vi "IVCharacterization.vi"() -> ()   [LabVIEW 2020]
panel:
  in  "循环":bool
  in  "参数值":dbl[](array[numeric])
  in  "负向扫描":bool
  in  "正向扫描":bool
  out "参数":string[](array[string])
  in  "Y轴":u16(ring)=2 items=["Time", "Voltage", "Current", "Real V"]
  in  "X轴":u16(ring)=1 items=["Time", "Voltage", "Current", "Real V"]
  out "XY图":picture
  in  "log":bool
  in  "缓冲区数据内容":u16(ring) items=["SET", "RESET", "TIME", "PSET", "PRESET"]
  out "缓存数据":bool
  in  "清除缓存数据":bool
  in  "功能选择":u16(ring)=1 items=["I-V扫描", "脉冲测试", "维持时间"]
  in  "4-wire":bool
  in  "自行输入nplc":bool
  in  "时序优先":bool
  in  "测试人员":string
  in  "衬底":string(combo)
  in  "阻变物质":string(combo)
  in  "保存数据":bool
  in  "停止":bool
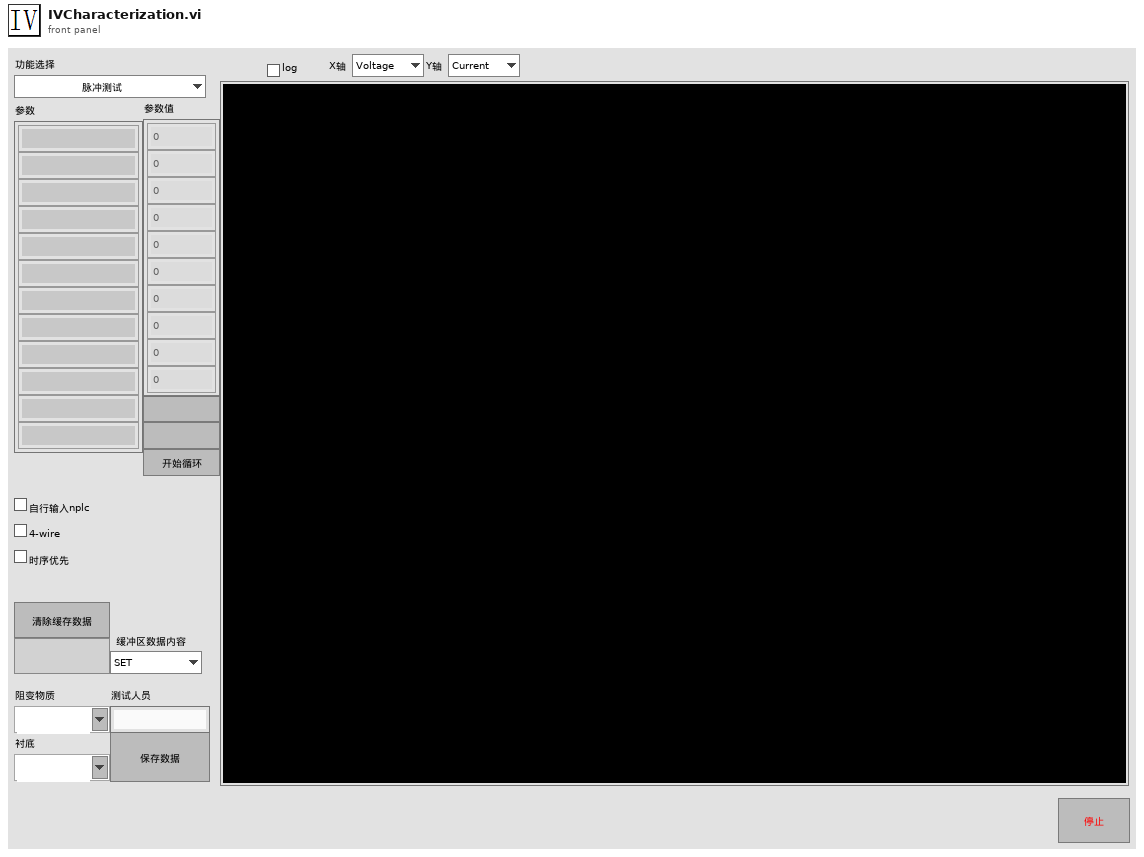
[diagram p1: front panel]
types:
  T1 = cluster{"nplc":dbl, "时序优先":bool, "时间点(ms)":dbl, "电压改变量":dbl, "极限电流(mA)":dbl, "扫描电压(V)":dbl, "4-wire ":bool}
  T2 = cluster{"nplc":dbl, "脉冲宽度(ms)":dbl, "读取电压":dbl, "极限电流(mA)":dbl, "脉冲电压(V)":dbl, "4-wire":bool, "读取次数":dbl}
  T3 = cluster{"nplc":dbl, "4-wire":bool, "读取间隔(ms)":dbl, "读取数量":dbl, "极限电流(mA)":dbl, "读取电压(V)":dbl}
  T4 = cluster{"测试人员":string, "阻变物质":string, "衬底":string}
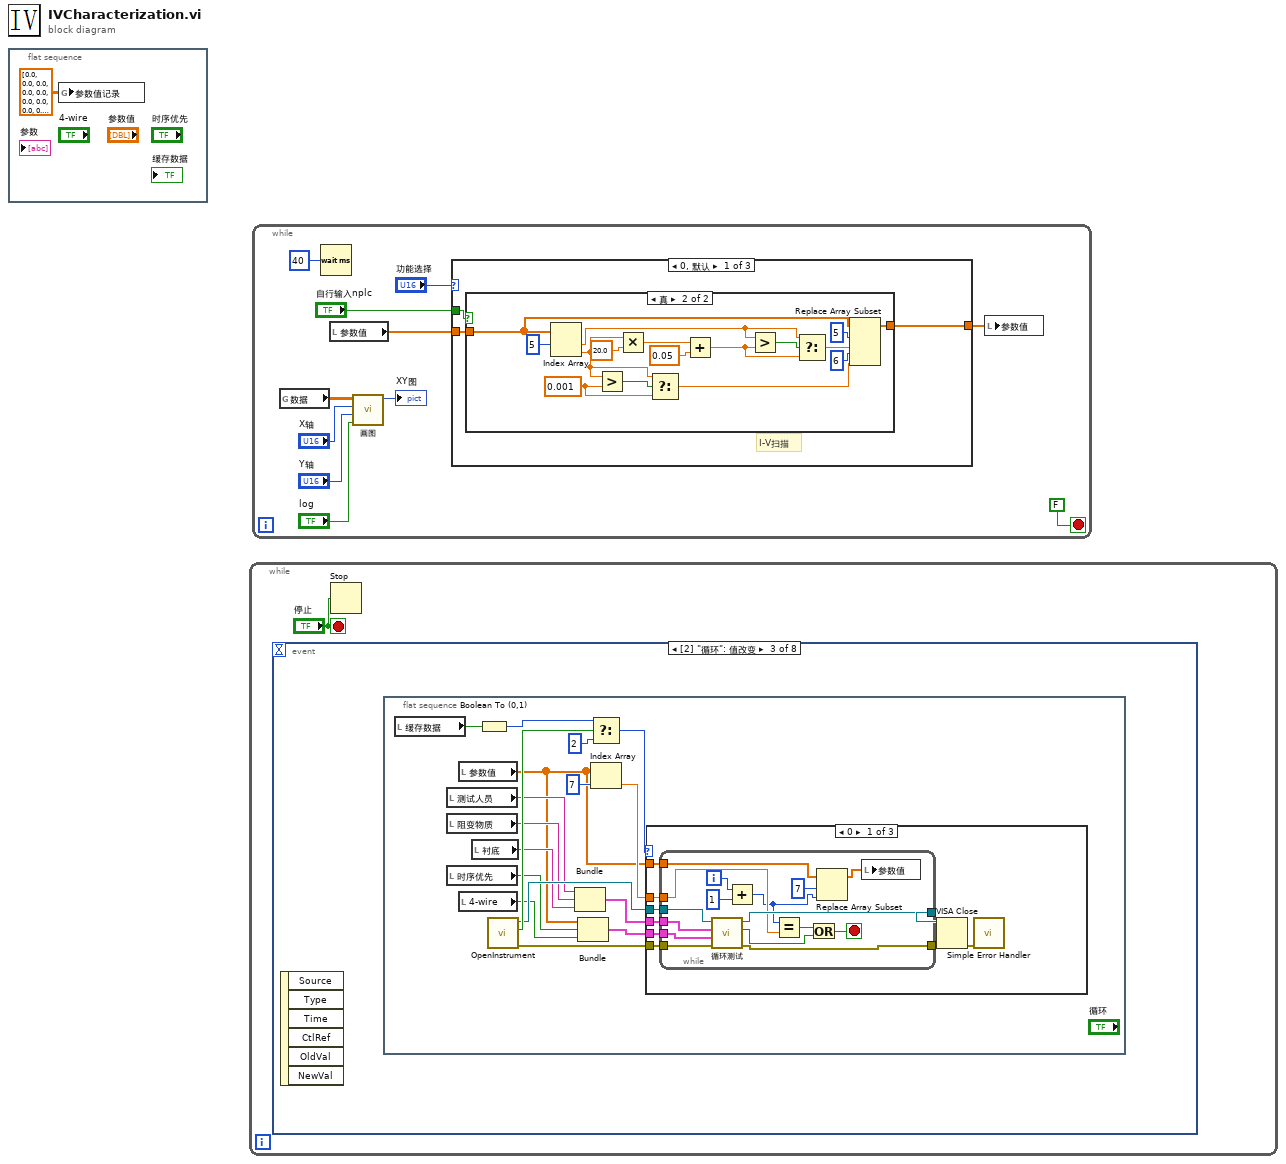
[diagram p0: block diagram]
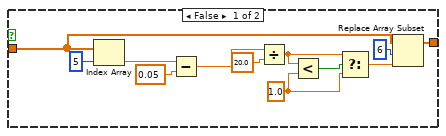
[diagram p2: hidden frame]
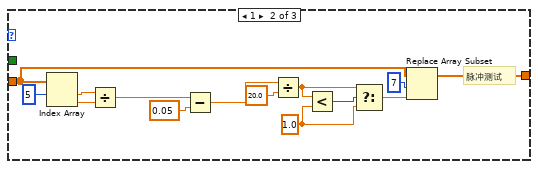
[diagram p3: hidden frame]
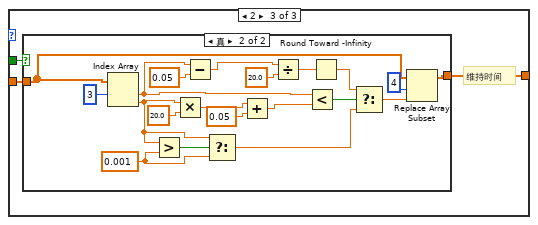
[diagram p4: hidden frame]
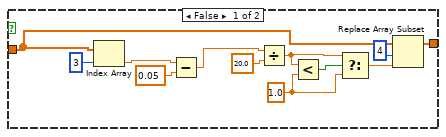
[diagram p5: hidden frame]
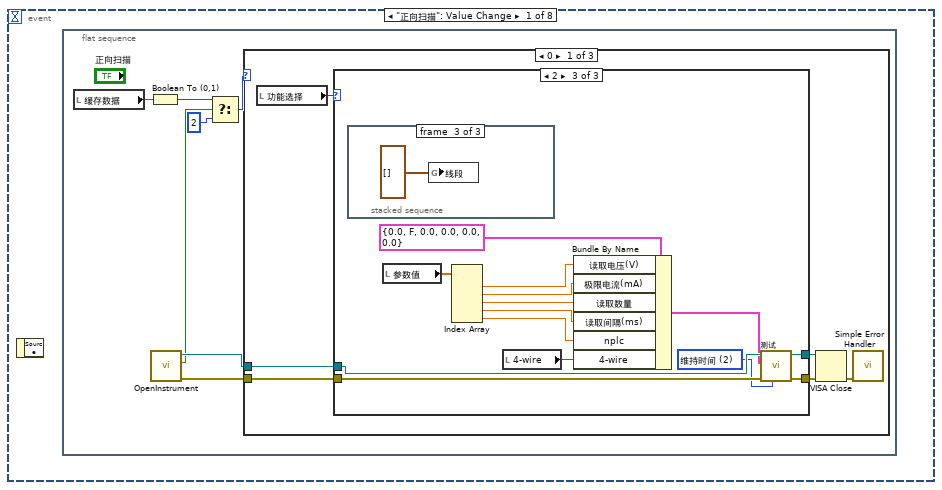
[diagram p6: hidden frame]
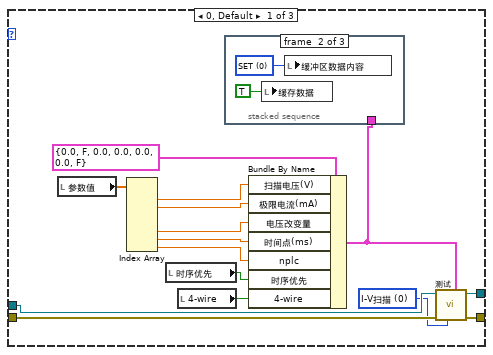
[diagram p7: hidden frame]
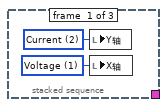
[diagram p8: hidden frame]
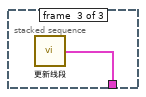
[diagram p9: hidden frame]
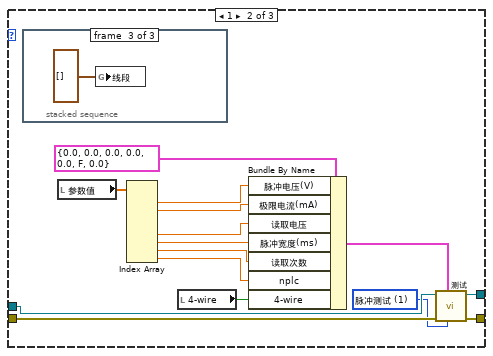
[diagram p10: hidden frame]
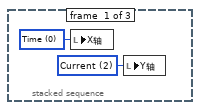
[diagram p11: hidden frame]
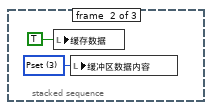
[diagram p12: hidden frame]
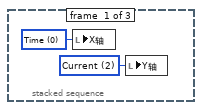
[diagram p13: hidden frame]
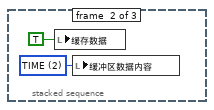
[diagram p14: hidden frame]
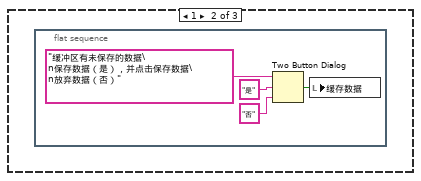
[diagram p15: hidden frame]
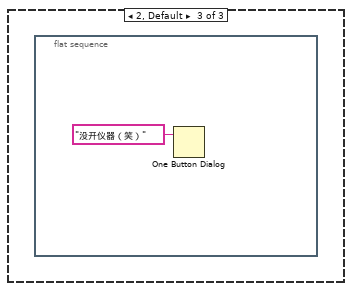
[diagram p16: hidden frame]
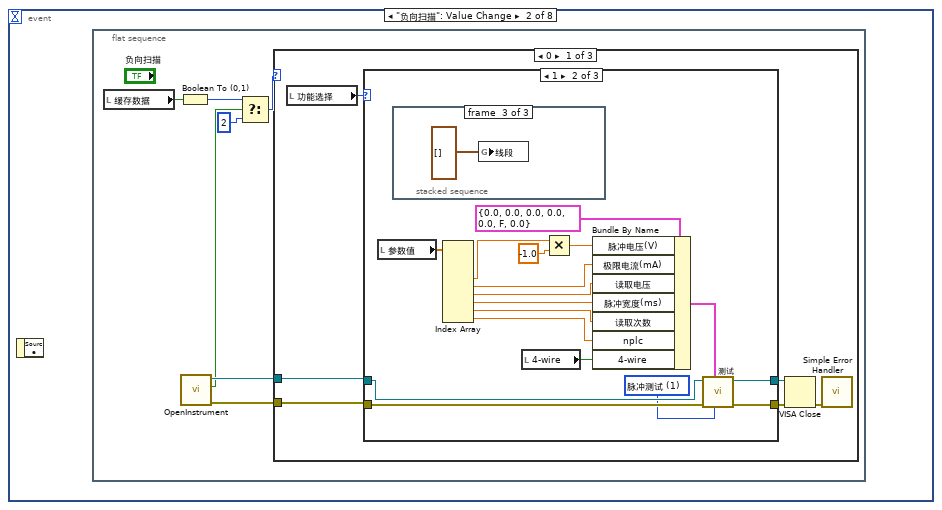
[diagram p17: hidden frame]
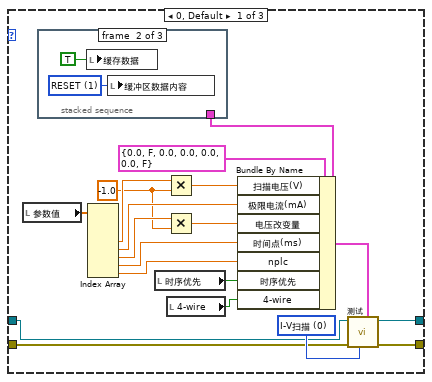
[diagram p18: hidden frame]
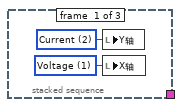
[diagram p19: hidden frame]
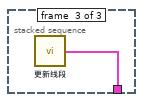
[diagram p20: hidden frame]
diagram:
  n1 = flat-sequence {
    frame #0 {
      n2 = global write "Global variable.vi" "参数值记录"(dbl[][] [[0.0, 0.0, 0.0, 0.0, 0.0, 0.0, 0.0, 0.0, 0.0, 0.0, 0.0, 0.0, 0.0, 0.0, 0.0, 0.0, 0.0, 0.0], [0.0, 0.0, 0.0, 0.0, 0.0, 0.0, 0.0, 0.0, 0.0, 0.0, 0.0, 0.0, 0.0, 0.0, 0.0, 0.0, 0.0, 0.0], [0.0, 0.0, 0.0, 0.0, 0.0, 0.0, 0.0, 0.0, 0.0, 0.0, 0.0, 0.0, 0.0, 0.0, 0.0, 0.0, 0.0, 0.0], [0.0, 0.0, 0.0, 0.0, 0.0, 0.0, 0.0, 0.0, 0.0, 0.0, 0.0, 0.0, 0.0, 0.0, 0.0, 0.0, 0.0, 0.0], [0.0, 0.0, 0.0, 0.0, 0.0, 0.0, 0.0, 0.0, 0.0, 0.0, 0.0, 0.0, 0.0, 0.0, 0.0, 0.0, 0.0, 0.0], [0.0, 0.0, 0.0, 0.0, 0.0, 0.0, 0.0, 0.0, 0.0, 0.0, 0.0, 0.0, 0.0, 0.0, 0.0, 0.0, 0.0, 0.0], [0.0, 0.0, 0.0, 0.0, 0.0, 0.0, 0.0, 0.0, 0.0, 0.0, 0.0, 0.0, 0.0, 0.0, 0.0, 0.0, 0.0, 0.0], [0.0, 0.0, 0.0, 0.0, 0.0, 0.0, 0.0, 0.0, 0.0, 0.0, 0.0, 0.0, 0.0, 0.0, 0.0, 0.0, 0.0, 0.0], [0.0, 0.0, 0.0, 0.0, 0.0, 0.0, 0.0, 0.0, 0.0, 0.0, 0.0, 0.0, 0.0, 0.0, 0.0, 0.0, 0.0, 0.0], [0.0, 0.0, 0.0, 0.0, 0.0, 0.0, 0.0, 0.0, 0.0, 0.0, 0.0, 0.0, 0.0, 0.0, 0.0, 0.0, 0.0, 0.0], [0.0, 0.0, 0.0, 0.0, 0.0, 0.0, 0.0, 0.0, 0.0, 0.0, 0.0, 0.0, 0.0, 0.0, 0.0, 0.0, 0.0, 0.0], [0.0, 0.0, 0.0, 0.0, 0.0, 0.0, 0.0, 0.0, 0.0, 0.0, 0.0, 0.0, 0.0, 0.0, 0.0, 0.0, 0.0, 0.0], [0.0, 0.0, 0.0, 0.0, 0.0, 0.0, 0.0, 0.0, 0.0, 0.0, 0.0, 0.0, 0.0, 0.0, 0.0, 0.0, 0.0, 0.0], [0.0, 0.0, 0.0, 0.0, 0.0, 0.0, 0.0, 0.0, 0.0, 0.0, 0.0, 0.0, 0.0, 0.0, 0.0, 0.0, 0.0, 0.0], [0.0, 0.0, 0.0, 0.0, 0.0, 0.0, 0.0, 0.0, 0.0, 0.0, 0.0, 0.0, 0.0, 0.0, 0.0, 0.0, 0.0, 0.0], [0.0, 0.0, 0.0, 0.0, 0.0, 0.0, 0.0, 0.0, 0.0, 0.0, 0.0, 0.0, 0.0, 0.0, 0.0, 0.0, 0.0, 0.0], [0.0, 0.0, 0.0, 0.0, 0.0, 0.0, 0.0, 0.0, 0.0, 0.0, 0.0, 0.0, 0.0, 0.0, 0.0, 0.0, 0.0, 0.0]]) -> ()
    }
  }
  n3 = while {
    stop <- "停止" stop-if-true
    n4 = event "事件结构" shown="[2] \"循环\": 值改变" {
      selector: _ -> [_ _ _ _ _ _ _ _]
      dyn-events: _ -> [_ _ _ _ _ _ _ _]
      timeout: _ -> [_ _ _ _ _ _ _ _]
      event "正向扫描": Value Change {
        n5 = event-data() -> ()  [unwired: 1 in, 1 out]
        n6 = flat-sequence {
          frame #0 {
            n7 = local read "缓存数据"() -> (w7:bool)
            n8 = Boolean To (0,1)(Boolean=w7) -> (0, 1=w5:i16)
            n9 = call "OpenInstrument.vi"() -> ("错误输出"=w9:errorcluster, "仪器存在"=w6:bool, "VISA资源名称输出"=w8:refnum<visa-resource-name>)  [unwired: 9 in]
            n10 = Select(t=w5, s=w6, f=i16 2) -> (s? t:f=w4:i16)
            n11 = case shown="0" w4 {
              tunnel: w9 -> [w11 _ _]
              tunnel: w8 -> [w10 _ _]
              frame 0 {
                n12 = local read "功能选择"() -> (w15:u16)
                n13 = case shown="2" w15 {
                  tunnel: w10 -> [w30 w50 w66]
                  tunnel: [w29 w48 w67] -> w12
                  tunnel: [w28 w47 w68] -> w13
                  tunnel: w11 -> [w27 w49 w69]
                  frame 0, Default {
                    w17 = u16 0 items=["I-V扫描", "脉冲测试", "维持时间"] ("功能选择")
                    n14 = local read "参数值"() -> (w23:dbl[])
                    n15 = Index Array(array=w23) -> (element #1=w22:dbl, element #2=w21:dbl, element #5=w20:dbl, element #6=w19:dbl, element #7=w18:dbl)  [unwired: 7 in, 2 out]
                    n16 = local read "时序优先"() -> (w25:bool)
                    n17 = local read "4-wire"() -> (w24:bool)
                    n18 = Bundle By Name(cluster=T1 {"nplc"=0.0, "时序优先"=FALSE, "时间点(ms)"=0.0, "电压改变量"=0.0, "极限电流(mA)"=0.0, "扫描电压(V)"=0.0, "4-wire "=FALSE} ("参数"), "扫描电压(V)"=w22, "极限电流(mA)"=w21, "电压改变量"=w20, "时间点(ms)"=w19, "nplc"=w18, "时序优先"=w25, "4-wire"=w24) -> (w16:T1)
                    n19 = stacked-sequence {
                      tunnel: w16 -> [_ _ w35]
                      frame #0 {
                        w31 = u16 2 items=["Time", "Voltage", "Current"] ("X轴")
                        w32 = u16 1 items=["Time", "Voltage", "Current"] ("X轴")
                        n20 = local write "Y轴"(w31) -> ()
                        n21 = local write "X轴"(w32) -> ()
                      }
                      frame #1 {
                        w34 = u16 0 items=["SET", "RESET", "TIME"] ("缓冲区数据内容")
                        n22 = local write "缓存数据"(TRUE) -> ()
                        n23 = local write "缓冲区数据内容"(w34) -> ()
                      }
                      frame #2 {
                        n24 = call "更新线段.vi"("参数"=w35) -> ()
                      }
                    }
                    n25 = call "测试.vi"("I-V扫描"=w16, "功能选择"=w17, "错误输入"=w27, "VISA资源名称"=w30) -> ("错误输出"=w28:errorcluster, "VISA资源名称输出"=w29:refnum<visa-resource-name>)  [unwired: 6 in]
                  }
                  frame 1 {
                    w37 = u16 1 items=["I-V扫描", "脉冲测试", "维持时间"] ("功能选择")
                    n26 = stacked-sequence {
                      frame #0 {
                        w51 = u16 2 items=["Time", "Voltage", "Current"] ("X轴")
                        w52 = u16 0 items=["Time", "Voltage", "Current"] ("X轴")
                        n27 = local write "X轴"(w52) -> ()
                        n28 = local write "Y轴"(w51) -> ()
                      }
                      frame #1 {
                        w54 = u16 3 items=["SET", "RESET", "TIME", "Pset", "Preset"] ("缓冲区数据内容")
                        n29 = local write "缓存数据"(TRUE ("缓存数据")) -> ()
                        n30 = local write "缓冲区数据内容"(w54) -> ()
                      }
                      frame #2 {
                        n31 = global write "Global variable.vi" "线段"(cluster{i32, i32}[] [] ("线段")) -> ()
                      }
                    }
                    n32 = local read "参数值"() -> (w44:dbl[])
                    n33 = Index Array(array=w44) -> (element #1=w43:dbl, element #2=w42:dbl, element #5=w41:dbl, element #6=w40:dbl, element #7=w39:dbl, element #8=w38:dbl)  [unwired: 8 in, 2 out]
                    n34 = local read "4-wire"() -> (w45:bool)
                    n35 = Bundle By Name(cluster=T2 {"nplc"=0.0, "脉冲宽度(ms)"=0.0, "读取电压"=0.0, "极限电流(mA)"=0.0, "脉冲电压(V)"=0.0, "4-wire"=FALSE, "读取次数"=0.0} ("脉冲测试"), "脉冲电压(V)"=w43, "极限电流(mA)"=w42, "读取电压"=w41, "脉冲宽度(ms)"=w40, "读取次数"=w39, "nplc"=w38, "4-wire"=w45) -> (w36:T2)
                    n36 = call "测试.vi"("功能选择"=w37, "脉冲测试"=w36, "错误输入"=w49, "VISA资源名称"=w50) -> ("错误输出"=w47:errorcluster, "VISA资源名称输出"=w48:refnum<visa-resource-name>)  [unwired: 6 in]
                  }
                  frame 2 {
                    w56 = u16 2 items=["I-V扫描", "脉冲测试", "维持时间"] ("功能选择")
                    n37 = stacked-sequence {
                      frame #0 {
                        w70 = u16 2 items=["Time", "Voltage", "Current"] ("X轴")
                        w71 = u16 0 items=["Time", "Voltage", "Current"] ("X轴")
                        n38 = local write "X轴"(w71) -> ()
                        n39 = local write "Y轴"(w70) -> ()
                      }
                      frame #1 {
                        w73 = u16 2 items=["SET", "RESET", "TIME"] ("缓冲区数据内容")
                        n40 = local write "缓存数据"(TRUE ("正标记")) -> ()
                        n41 = local write "缓冲区数据内容"(w73) -> ()
                      }
                      frame #2 {
                        n42 = global write "Global variable.vi" "线段"(cluster{i32, i32}[] [] ("线段")) -> ()
                      }
                    }
                    n43 = local read "参数值"() -> (w65:dbl[])
                    n44 = Index Array(array=w65) -> (element #1=w63:dbl, element #2=w62:dbl, element #3=w61:dbl, element #4=w60:dbl, element #5=w59:dbl)  [unwired: 5 in]
                    n45 = local read "4-wire"() -> (w58:bool)
                    n46 = Bundle By Name(cluster=T3 {"nplc"=0.0, "4-wire"=FALSE, "读取间隔(ms)"=0.0, "读取数量"=0.0, "极限电流(mA)"=0.0, "读取电压(V)"=0.0} ("参数"), "读取电压(V)"=w63, "极限电流(mA)"=w62, "读取数量"=w61, "读取间隔(ms)"=w60, "nplc"=w59, "4-wire"=w58) -> (w57:T3)
                    n47 = call "测试.vi"("功能选择"=w56, "错误输入"=w69, "维持时间"=w57, "VISA资源名称"=w66) -> ("错误输出"=w68:errorcluster, "VISA资源名称输出"=w67:refnum<visa-resource-name>)  [unwired: 6 in]
                  }
                }
                n48 = VISA Close(VISA resource name=w12, error in (no error)=w13) -> (error out=w14:errorcluster)
                n49 = call <vilib>:"Simple Error Handler.vi"("error in (no error)"=w14) -> ()  [unwired: 4 in, 5 out]
              }
              frame 1 {
                n50 = flat-sequence {
                  frame #0 {
                    n51 = Two Button Dialog(message="缓冲区有未保存的数据\n保存数据（是），并点击保存数据\n放弃数据（否）" ("消息"), 1:"否" ("F按钮名称（“取消”）"), 2:"是" ("T按钮名称（“确定”）")) -> (T button?=w75:bool)
                    n52 = local write "缓存数据"(w75) -> ()
                  }
                }
              }
              frame 2, Default {
                n53 = flat-sequence {
                  frame #0 {
                    n54 = One Button Dialog(message="没开仪器（笑）" ("消息")) -> ()  [unwired: 1 in, 1 out]
                  }
                }
              }
            }
          }
        }
      }
      event "负向扫描": Value Change {
        n55 = event-data() -> ()  [unwired: 1 in, 1 out]
        n56 = flat-sequence {
          frame #0 {
            n57 = local read "缓存数据"() -> (w81:bool)
            n58 = Boolean To (0,1)(Boolean=w81) -> (0, 1=w84:i16)
            n59 = call "OpenInstrument.vi"() -> ("错误输出"=w86:errorcluster, "仪器存在"=w82:bool, "VISA资源名称输出"=w85:refnum<visa-resource-name>)  [unwired: 9 in]
            n60 = Select(t=w84, s=w82, f=i16 2) -> (s? t:f=w80:i16)
            n61 = case shown="0" w80 {
              tunnel: w86 -> [w88 _ _]
              tunnel: w85 -> [w87 _ _]
              frame 0 {
                n62 = local read "功能选择"() -> (w92:u16)
                n63 = case shown="1" w92 {
                  tunnel: w87 -> [w94 w129 w139]
                  tunnel: [w110 w127 w139] -> w89
                  tunnel: [w109 w126 w138] -> w90
                  tunnel: w88 -> [w95 w128 w138]
                  frame 0, Default {
                    w97 = -1.0 ("y")
                    w96 = u16 0 items=["I-V扫描", "脉冲测试", "维持时间"] ("功能选择")
                    n64 = local read "参数值"() -> (w103:dbl[])
                    n65 = Index Array(array=w103) -> (element #3=w102:dbl, element #4=w101:dbl, element #5=w100:dbl, element #6=w99:dbl, element #7=w98:dbl)  [unwired: 7 in, 2 out]
                    n66 = local read "时序优先"() -> (w107:bool)
                    n67 = Multiply(x=w102, y=w97) -> (x*y=w105:dbl)
                    n68 = Multiply(x=w100, y=w97) -> (x*y=w104:dbl)
                    n69 = local read "4-wire"() -> (w106:bool)
                    n70 = Bundle By Name(cluster=T1 {"nplc"=0.0, "时序优先"=FALSE, "时间点(ms)"=0.0, "电压改变量"=0.0, "极限电流(mA)"=0.0, "扫描电压(V)"=0.0, "4-wire "=FALSE} ("参数"), "扫描电压(V)"=w105, "极限电流(mA)"=w101, "电压改变量"=w104, "时间点(ms)"=w99, "nplc"=w98, "时序优先"=w107, "4-wire"=w106) -> (w93:T1)
                    n71 = stacked-sequence {
                      tunnel: w93 -> [_ _ w115]
                      frame #0 {
                        w111 = u16 2 items=["Time", "Voltage", "Current"] ("X轴")
                        w112 = u16 1 items=["Time", "Voltage", "Current"] ("X轴")
                        n72 = local write "Y轴"(w111) -> ()
                        n73 = local write "X轴"(w112) -> ()
                      }
                      frame #1 {
                        w114 = u16 1 items=["SET", "RESET", "TIME"] ("缓冲区数据内容")
                        n74 = local write "缓存数据"(TRUE) -> ()
                        n75 = local write "缓冲区数据内容"(w114) -> ()
                      }
                      frame #2 {
                        n76 = call "更新线段.vi"("参数"=w115) -> ()
                      }
                    }
                    n77 = call "测试.vi"("I-V扫描"=w93, "功能选择"=w96, "错误输入"=w95, "VISA资源名称"=w94) -> ("错误输出"=w109:errorcluster, "VISA资源名称输出"=w110:refnum<visa-resource-name>)  [unwired: 6 in]
                  }
                  frame 1 {
                    w117 = u16 1 items=["I-V扫描", "脉冲测试", "维持时间"] ("功能选择")
                    n78 = local read "参数值"() -> (w130:dbl[])
                    n79 = stacked-sequence {
                      frame #0 {
                        w133 = u16 2 items=["Time", "Voltage", "Current"] ("X轴")
                        w134 = u16 0 items=["Time", "Voltage", "Current"] ("X轴")
                        n80 = local write "X轴"(w134) -> ()
                        n81 = local write "Y轴"(w133) -> ()
                      }
                      frame #1 {
                        w136 = u16 4 items=["SET", "RESET", "TIME", "Pset", "Preset"] ("缓冲区数据内容")
                        n82 = local write "缓存数据"(TRUE ("缓存数据")) -> ()
                        n83 = local write "缓冲区数据内容"(w136) -> ()
                      }
                      frame #2 {
                        n84 = global write "Global variable.vi" "线段"(cluster{i32, i32}[] [] ("线段")) -> ()
                      }
                    }
                    n85 = Index Array(array=w130) -> (element #3=w123:dbl, element #4=w122:dbl, element #5=w121:dbl, element #6=w120:dbl, element #7=w119:dbl, element #8=w118:dbl)  [unwired: 8 in, 2 out]
                    n86 = local read "4-wire"() -> (w131:bool)
                    n87 = Multiply(x=w123, y=-1.0) -> (x*y=w124:dbl)
                    n88 = Bundle By Name(cluster=T2 {"nplc"=0.0, "脉冲宽度(ms)"=0.0, "读取电压"=0.0, "极限电流(mA)"=0.0, "脉冲电压(V)"=0.0, "4-wire"=FALSE, "读取次数"=0.0} ("脉冲测试"), "脉冲电压(V)"=w124, "极限电流(mA)"=w122, "读取电压"=w121, "脉冲宽度(ms)"=w120, "读取次数"=w119, "nplc"=w118, "4-wire"=w131) -> (w116:T2)
                    n89 = call "测试.vi"("功能选择"=w117, "脉冲测试"=w116, "错误输入"=w128, "VISA资源名称"=w129) -> ("错误输出"=w126:errorcluster, "VISA资源名称输出"=w127:refnum<visa-resource-name>)  [unwired: 6 in]
                  }
                  frame 2 {
                  }
                }
                n90 = VISA Close(VISA resource name=w89, error in (no error)=w90) -> (error out=w91:errorcluster)
                n91 = call <vilib>:"Simple Error Handler.vi"("error in (no error)"=w91) -> ()  [unwired: 4 in, 5 out]
              }
              frame 1 {
                n92 = flat-sequence {
                  frame #0 {
                    n93 = Two Button Dialog(message="缓冲区有未保存的数据\n保存数据（是），并点击保存数据\n放弃数据（否）" ("消息"), 1:"否" ("F按钮名称（“取消”）"), 2:"是" ("T按钮名称（“确定”）")) -> (T button?=w140:bool)
                    n94 = local write "缓存数据"(w140) -> ()
                  }
                }
              }
              frame 2, Default {
                n95 = flat-sequence {
                  frame #0 {
                    n96 = One Button Dialog(message="没开仪器（笑）" ("消息")) -> ()  [unwired: 1 in, 1 out]
                  }
                }
              }
            }
          }
        }
      }
      event "循环": Value Change {
        n97 = event-data() -> ()  [unwired: 1 in, 6 out]
        n98 = flat-sequence {
          frame #0 {
            n99 = local read "缓存数据"() -> (w158:bool)
            n100 = local read "测试人员"() -> (w154:string)
            n101 = local read "阻变物质"() -> (w153:string)
            n102 = local read "时序优先"() -> (w150:bool)
            n103 = local read "参数值"() -> (w145:dbl[])
            n104 = local read "4-wire"() -> (w149:bool)
            n105 = local read "衬底"() -> (w152:string)
            n106 = Boolean To (0,1)(Boolean=w158) -> (0, 1=w160:i16)
            n107 = call "OpenInstrument.vi"() -> ("错误输出"=w156:errorcluster, "仪器存在"=w161:bool, "VISA资源名称输出"=w157:refnum<visa-resource-name>)  [unwired: 9 in]
            n108 = Bundle("测试人员"=w154, "阻变物质"=w153, "衬底"=w152) -> (w151:T4)  [unwired: 1 in]
            n109 = Bundle("参数值"=w145, "时序优先"=w150, "4-wire"=w149) -> (w148:cluster{"参数值":dbl[], "时序优先":bool, "4-wire":bool})  [unwired: 1 in]
            n110 = Select(t=w160, s=w161, f=i16 2) -> (s? t:f=w155:i16)
            n111 = Index Array(array=w145, index=7 ("索引")) -> (element=w146:dbl)
            n112 = case shown="0" w155 {
              tunnel: w157 -> [w169 _ _]
              tunnel: w156 -> [w168 _ _]
              tunnel: w151 -> [w165 _ _]
              tunnel: w148 -> [w164 _ _]
              tunnel: w146 -> [w163 _ _]
              tunnel: w145 -> [w162 _ _]
              frame 0 {
                n113 = while {
                  tunnel: w169 -> [w186]
                  tunnel: w168 -> [w185]
                  tunnel: [w184] -> w167
                  tunnel: [w183] -> w166
                  tunnel: w165 -> [w182]
                  tunnel: w164 -> [w181]
                  tunnel: w163 -> [w178]
                  tunnel: w162 -> [w174]
                  i -> [w180]
                  stop <- w175 stop-if-true
                  n114 = call "循环测试.vi"("错误输入"=w185, "测试参数"=w181, "保存参数"=w182, "VISA资源名称"=w186) -> ("错误输出"=w183:errorcluster, "循环未完成"=w176:bool, "VISA资源名称输出"=w184:refnum<visa-resource-name>)  [unwired: 5 in]
                  n115 = Add(x=w180, y=1) -> (x+y=w172:i32)
                  n116 = Equal?(x=w172, y=w178) -> (x = y?=w177:bool)
                  n117 = Or(x=w177, y=w176) -> (x .or. y?=w175:bool)
                  n118 = Replace Array Subset(array=w174, new element=w172, index=7 ("索引")) -> (w171:dbl[])
                  n119 = local write "参数值"(w171) -> ()
                }
                n120 = VISA Close(VISA resource name=w167, error in (no error)=w166) -> (error out=w170:errorcluster)
                n121 = call <vilib>:"Simple Error Handler.vi"("error in (no error)"=w170) -> ()  [unwired: 4 in, 5 out]
              }
              frame 1 {
                n122 = flat-sequence {
                  frame #0 {
                    n123 = Two Button Dialog(message="缓冲区有未保存的数据\n保存数据（是），并点击保存数据\n放弃数据（否）" ("消息"), 1:"否" ("F按钮名称（“取消”）"), 2:"是" ("T按钮名称（“确定”）")) -> ()  [unwired: 1 out]
                  }
                }
              }
              frame 2, Default {
                n124 = flat-sequence {
                  frame #0 {
                    n125 = One Button Dialog(message="没开仪器（笑）" ("消息")) -> ()  [unwired: 1 in, 1 out]
                  }
                }
              }
            }
          }
        }
      }
      event "功能选择": Value Change {
        n126 = event-data() -> ("NewVal"=w191:u16)  [unwired: 1 in]
        n127 = flat-sequence {
          tunnel: w191 -> [w193]
          frame #0 {
            n128 = case shown="0, 默认" w193 {
              tunnel: [string[] ["正向扫描电压(V)", "正向极限电流(mA)", "反向扫描电压(V)", "反向极限电流(mA)", "电压改变量", "维持时间(ms)", "nplc", "循环次数", "", "", "正向扫描", "负向扫描"] string[] ["正向脉冲电压(V)", "正向极限电流(mA)", "负向脉冲电压(V)", "负向极限电流(mA)", "读取电压", "脉冲宽度(ms)", "读取次数", "nplc", "", "", "正向脉冲", "负向脉冲"] string[] ["读取电压(V)", "极限电流(mA)", "读取数量", "读取间隔(ms)", "nplc", "", "", "", "", "", "开始测试"]] -> w192
              frame 0, Default {
              }
              frame 1 {
              }
              frame 2 {
              }
            }
            n129 = local write "参数"(w192) -> ()
            n130 = case shown="0, 默认" w193 {
              tunnel: [dbl[] [1.0, 1.0, 1.0, 1.0, 0.01, 25.0, 0.0, 10.0] dbl[] [1.0, 2.0, 1.0, 2.0, 0.1, 20.0, 200.0, 0.0025] dbl[] [0.1, 1.0, 100.0, 100.0, 1.0]] -> w194
              frame 0, Default {
              }
              frame 1 {
              }
              frame 2 {
              }
            }
            n131 = global read "Global variable.vi" "参数值记录"() -> (w206:dbl[][])
            n132 = Array Size(array=w194) -> (size(s)=w204:i32)
            n133 = Array Subset(array=w206, index (row)=0 ("索引"), length (row)=w204, index (col)=w193, length (col)=1 ("长度")) -> (w202:dbl[][])
            n134 = Index Array(array=w202, index (col)=0 ("索引 (行)")) -> (element=w196:dbl[])  [unwired: 1 in]
            n135 = Index Array(array=w196, index=0 ("索引")) -> (element=w199:dbl)
            n136 = Equal?(x=w199, y=0.0) -> (x = y?=w197:bool)
            n137 = Select(t=w194, s=w197, f=w196) -> (s? t:f=w195:dbl[])
            n138 = local write "参数值"(w195) -> ()
          }
        }
      }
      event "参数值": Value Change {
        n139 = event-data() -> ("OldVal"=w214:dbl[], "NewVal"=w213:dbl[])  [unwired: 1 in]
        n140 = flat-sequence {
          tunnel: w214 -> [w223]
          tunnel: w213 -> [w219]
          frame #0 {
            n141 = Equal?(x=w223, y=w219) -> (x = y?=w222:bool[])
            n142 = local read "功能选择"() -> (w215:u16)
            n143 = Search 1D Array(1D array=w222, element=FALSE ("元素")) -> (index of element=w220:i32)  [unwired: 1 in]
            n144 = case shown="1" w215 {
              tunnel: w220 -> [_ w227]
              tunnel: w219 -> [w224 w226]
              tunnel: [w224 w225] -> w217
              frame 0, Default {
              }
              frame 1 {
                n145 = case shown="5" w227 {
                  selector: w227 -> [_ w236]
                  tunnel: w226 -> [w228 w233]
                  tunnel: [w228 w229] -> w225
                  frame 0, Default {
                  }
                  frame 5 {
                    n146 = Index Array(array=w233, index=w236) -> (element=w235:dbl)
                    n147 = Divide(x=w235, y=0.07) -> (x/y=w231:dbl)
                    n148 = Round Toward -Infinity(1:w231) -> (0:w230:dbl)
                    n149 = Replace Array Subset(array=w233, new element=w230, index=6 ("索引")) -> (w229:dbl[])
                  }
                }
              }
            }
            n150 = global read "Global variable.vi" "参数值记录"() -> (w218:dbl[][])
            n151 = local write "参数值"(w217) -> ()
            n152 = Replace Array Subset(array=w218, new element=w217, index (col)=w215) -> (w216:dbl[][])  [unwired: 1 in]
            n153 = global write "Global variable.vi" "参数值记录"(w216) -> ()
          }
        }
      }
      event "保存数据": Value Change {
        n154 = event-data() -> ()  [unwired: 1 in, 1 out]
        n155 = flat-sequence {
          frame #0 {
            n156 = flat-sequence {
              tunnel: [w238] -> w237
              frame #0 {
                n157 = local read "缓存数据"() -> (w238:bool)
              }
            }
            n158 = case shown="真" w237 {
              frame False {
              }
              frame True {
                n159 = case shown="1" "缓冲区数据内容" {
                  tunnel: ["SET" "RESET" "TIME" "PSET" "PRESET"] -> w251
                  tunnel: [1 3 1 1 3] -> w240
                  frame 0, Default {
                  }
                  frame 1 {
                  }
                  frame 2 {
                  }
                  frame 3 {
                  }
                  frame 4 {
                  }
                }
                n160 = local read "参数值"() -> (w242:dbl[])
                n161 = Index Array(array=w242, index=w240) -> (element=w241:dbl)
                n162 = global read "Global variable.vi" "时间标识"() -> (w249:timestamp)
                n163 = global read "Global variable.vi" "数据"() -> (w243:dbl[][])
                n164 = Format Into String(format string="%s-%s-%s-%.1f" ("格式字符串"), "阻变物质", "衬底", w251, w241) -> (resulting string=w247:string)  [unwired: 2 in, 1 out]
                n165 = call "Save Data.vi"("数据标记"=w247, "测试人员"="测试人员", "扫描数据"=w243, "时间标识"=w249) -> ("保存失败"=w244:bool)  [unwired: 7 in]
                n166 = local write "缓存数据"(w244) -> ()
              }
            }
          }
        }
      }
      event "清除缓存数据": Value Change {
        n167 = event-data() -> ()  [unwired: 1 in, 1 out]
        n168 = flat-sequence {
          frame #0 {
            n169 = call "OpenInstrument.vi"() -> ("错误输出"=w263:errorcluster, "仪器存在"=w262:bool, "VISA资源名称输出"=w264:refnum<visa-resource-name>)  [unwired: 9 in]
            n170 = case shown="真" w262 {
              tunnel: w264 -> [_ w268]
              tunnel: w263 -> [_ w267]
              frame False {
                n171 = One Button Dialog(message="没开仪器（笑）" ("消息")) -> ()  [unwired: 1 in, 1 out]
              }
              frame True {
                n172 = VISA Close(VISA resource name=w268, error in (no error)=w267) -> (error out=w266:errorcluster)
                n173 = call <vilib>:"Simple Error Handler.vi"("error in (no error)"=w266) -> ()  [unwired: 4 in, 5 out]
              }
            }
          }
        }
        n174 = flat-sequence {
          frame #0 {
            n175 = local write "缓存数据"(FALSE) -> ()
            n176 = global write "Global variable.vi" "数据"(dbl[][] [] ("数据")) -> ()
          }
        }
      }
      event "停止": Value Change {
        n177 = event-data() -> ()  [unwired: 1 in, 1 out]
      }
    }
    n178 = Stop(stop? (T)="停止") -> ()
  }
  n179 = while {
    stop <- FALSE stop-if-true
    n180 = global read "Global variable.vi" "数据"() -> (w271:dbl[][])
    n181 = Wait (ms)(milliseconds to wait=u32 40 ("等待时间（毫秒）")) -> ()  [unwired: 1 out]
    n182 = local read "参数值"() -> (w274:dbl[])
    n183 = call "画图.vi"("log"="log", "Y轴"="Y轴", "X轴"="X轴", "扫描数据"=w271) -> ("XY图"=→"XY图":picture)  [unwired: 7 in]
    n184 = case shown="0, 默认" "功能选择" {
      tunnel: "自行输入nplc" -> [w284 _ w328]
      tunnel: w274 -> [w283 w318 w329]
      tunnel: [w282 w317 w327] -> w273
      frame 0, Default {
        # "I-V扫描"
        n185 = case shown="真" w284 {
          tunnel: w283 -> [w290 w308]
          tunnel: [w289 w306] -> w282
          frame False {
            w286 = 1.0 ("y")
            n186 = Index Array(array=w290, index=5 ("索引")) -> (element=w293:dbl)
            n187 = Subtract(x=w293, y=0.05) -> (x-y=w295:dbl)
            n188 = Divide(x=w295, y=20.0) -> (x/y=w288:dbl)
            n189 = Less?(x=w288, y=w286) -> (x < y?=w287:bool)
            n190 = Select(t=w288, s=w287, f=w286) -> (s? t:f=w285:dbl)
            n191 = Replace Array Subset(array=w290, new element=w285, index=6 ("索引")) -> (w289:dbl[])
          }
          frame True {
            w298 = 0.001 ("y")
            n192 = Index Array(array=w308, index #1=5 ("索引")) -> (element #1=w304:dbl, element #2=w297:dbl)  [unwired: 1 in]
            n193 = Greater?(x=w297, y=w298) -> (0:w301:bool)
            n194 = Multiply(x=w297, y=20.0) -> (x*y=w311:dbl)
            n195 = Select(t=w297, s=w301, f=w298) -> (s? t:f=w299:dbl)
            n196 = Add(x=w311, y=0.05) -> (x+y=w303:dbl)
            n197 = Greater?(x=w304, y=w303) -> (0:w305:bool)
            n198 = Select(t=w304, s=w305, f=w303) -> (s? t:f=w302:dbl)
            n199 = Replace Array Subset(array=w308, new element #1=w302, index #1=5 ("索引"), new element #2=w299, index #2=6 ("索引")) -> (w306:dbl[])
          }
        }
      }
      frame 1 {
        w314 = 1.0 ("y")
        # "脉冲测试"
        n200 = Index Array(array=w318, index #1=5 ("索引")) -> (element #1=w321:dbl, element #2=w320:dbl)  [unwired: 1 in]
        n201 = Divide(x=w321, y=w320) -> (x/y=w319:dbl)
        n202 = Subtract(x=w319, y=0.05) -> (x-y=w325:dbl)
        n203 = Divide(x=w325, y=20.0) -> (x/y=w315:dbl)
        n204 = Less?(x=w315, y=w314) -> (x < y?=w316:bool)
        n205 = Select(t=w315, s=w316, f=w314) -> (s? t:f=w313:dbl)
        n206 = Replace Array Subset(array=w318, new element=w313, index=7 ("索引")) -> (w317:dbl[])
      }
      frame 2 {
        # "维持时间"
        n207 = case shown="真" w328 {
          tunnel: w329 -> [w335 w357]
          tunnel: [w334 w355] -> w327
          frame False {
            w331 = 1.0 ("y")
            n208 = Index Array(array=w335, index=3 ("索引")) -> (element=w338:dbl)
            n209 = Subtract(x=w338, y=0.05) -> (x-y=w340:dbl)
            n210 = Divide(x=w340, y=20.0) -> (x/y=w333:dbl)
            n211 = Less?(x=w333, y=w331) -> (x < y?=w332:bool)
            n212 = Select(t=w333, s=w332, f=w331) -> (s? t:f=w330:dbl)
            n213 = Replace Array Subset(array=w335, new element=w330, index=4 ("索引")) -> (w334:dbl[])
          }
          frame True {
            w344 = 0.001 ("y")
            n214 = Index Array(array=w357, index #1=3 ("索引")) -> (element #1=w350:dbl, element #2=w343:dbl)  [unwired: 1 in]
            n215 = Greater?(x=w343, y=w344) -> (0:w345:bool)
            n216 = Multiply(x=w343, y=20.0) -> (x*y=w360:dbl)
            n217 = Subtract(x=w350, y=0.05) -> (x-y=w352:dbl)
            n218 = Select(t=w343, s=w345, f=w344) -> (s? t:f=w342:dbl)
            n219 = Add(x=w360, y=0.05) -> (x+y=w346:dbl)
            n220 = Divide(x=w352, y=20.0) -> (x/y=w349:dbl)
            n221 = Less?(x=w350, y=w346) -> (x < y?=w347:bool)
            n222 = Round Toward -Infinity(1:w349) -> (0:w348:dbl)
            n223 = Select(t=w348, s=w347, f=w342) -> (s? t:f=w354:dbl)
            n224 = Replace Array Subset(array=w357, new element=w354, index=4 ("索引")) -> (w355:dbl[])
          }
        }
      }
    }
    n225 = local write "参数值"(w273) -> ()
  }
